vi "读取数据导入状态.vi"(8 "error in (no error)":errorcluster caption="错误输入（无错误）", 11 "抽取参数输入":refnum<class "抽取参数.lvclass">) -> (0 "error out":errorcluster caption="错误输出", 2 "数据导入状态":bool, 3 "抽取参数输出":refnum<class "抽取参数.lvclass">)   [LabVIEW 2020, in "抽取参数.lvclass"]
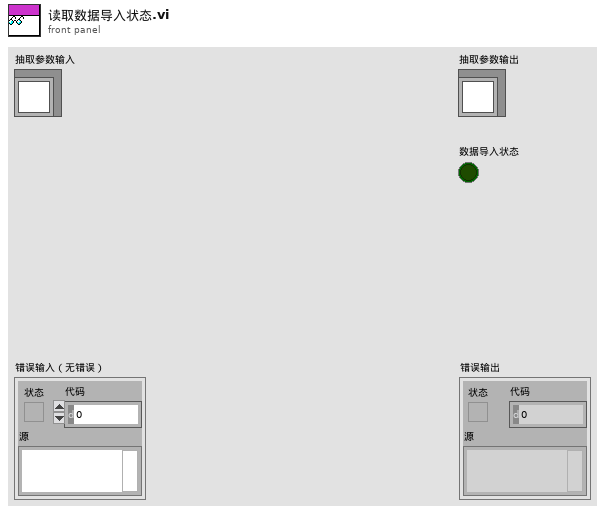
[diagram p1: front panel]
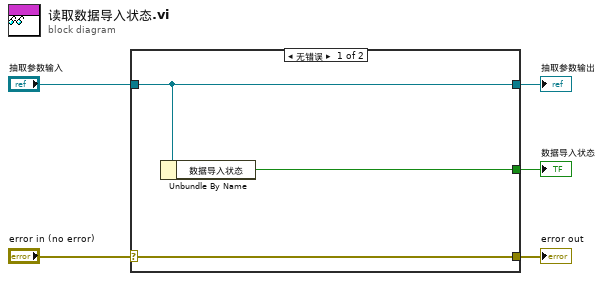
[diagram p0: block diagram]
diagram:
  n1 = case shown="无错误" "error in (no error)" {
    selector: "error in (no error)" -> [w8 w9]
    tunnel: [w8 w9] -> w4
    tunnel: [w7 w10] -> w2
    tunnel: "抽取参数输入" -> [w7 w10]
    tunnel: [w6 _] -> w1
    frame No Error {
      n2 = Unbundle By Name(w7) -> ("数据导入状态"=w6:bool)
    }
    frame Error {
    }
  }
  "error out" <- w4
  "抽取参数输出" <- w2
  "数据导入状态" <- w1
